vi "getSubSysAdapTestSetting.vi"() -> (3 "Test Setting":T1)   [LabVIEW 2016]
doc: "Get the test setting of SubSysAdap class."
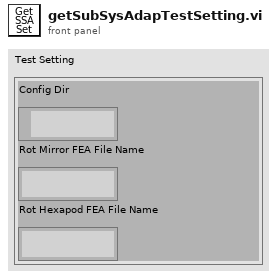
[diagram p1: front panel]
types:
  T1 = cluster{"Config Dir":path, "Rot Mirror FEA File Name":string, "Rot Hexapod FEA File Name":string}
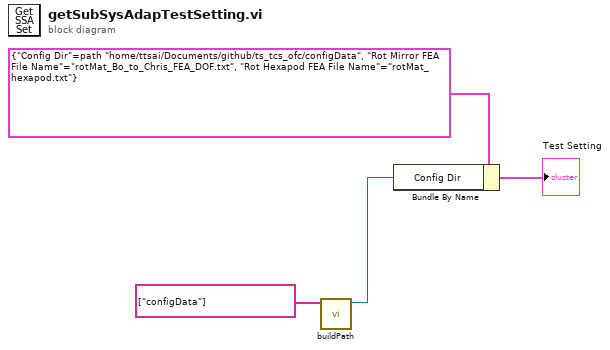
[diagram p0: block diagram]
diagram:
  n1 = call "buildPath.vi"("Path Name List"=string[] ["configData"]) -> ("New Path"=w4:path)  [unwired: 10 in]
  n2 = Bundle By Name(cluster=T1 {"Config Dir"=path "/home/ttsai/Documents/github/ts_tcs_ofc/configData", "Rot Mirror FEA File Name"="rotMat_Bo_to_Chris_FEA_DOF.txt", "Rot Hexapod FEA File Name"="rotMat_hexapod.txt"} ("Configuration"), "Config Dir"=w4) -> (→"Test Setting":T1)
